vi "Create.vi"(8 "error in (no error)":errorcluster, 9 "# Chans":i32, 10 "Size":i32, 11 "MsgQ":refnum<class "MessageQ.lvclass">) -> (0 "error out":errorcluster, 3 "Data Buffer out":refnum<class "Data Buffer.lvclass">)   [LabVIEW 2020, in "VolatusData.lvlib" / "Data Buffer.lvclass"]
uses:
  Data Buffer.lvclass
  Data Buffer.lvclass/Data Buffer.ctl
  Volatus/MessageQ/MessageQ.lvclass
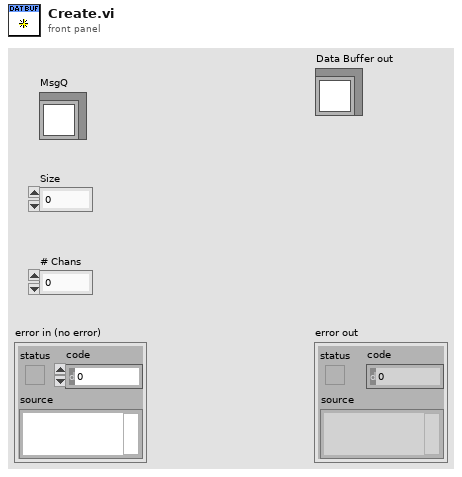
[diagram p1: front panel]
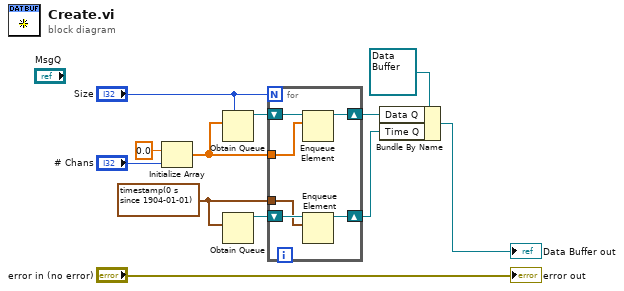
[diagram p0: block diagram]
diagram:
  w2 = timestamp(0 s since 1904-01-01)
  n1 = Initialize Array(0.0 ("element"), "# Chans") -> (w4:dbl[])
  n2 = Obtain Queue(max queue size (-1, unlimited)="Size", element data type=w4) -> (queue out=w9:refnum<queue>)  [unwired: 3 in, 2 out]
  n3 = Obtain Queue(element data type=w2) -> (queue out=w3:refnum<queue>)  [unwired: 4 in, 2 out]
  n4 = for {
    N: "Size" -> [_]
    shift-right: [w17] -> w6
    shift-left: w9 -> [w18]
    tunnel: w4 -> [w16]
    tunnel: w2 -> [w14]
    shift-right: [w13] -> w1
    shift-left: w3 -> [w15]
    n5 = Enqueue Element(queue=w18, element=w16) -> (queue out=w17:refnum<queue>)  [unwired: 2 in, 2 out]
    n6 = Enqueue Element(queue=w15, element=w14) -> (queue out=w13:refnum<queue>)  [unwired: 2 in, 2 out]
  }
  n7 = Bundle By Name(cluster=refnum<class "Data Buffer.lvclass"> refnum ("Data Buffer in"), "Data Q"=w6, "Time Q"=w1) -> (→"Data Buffer out":refnum<class "Data Buffer.lvclass">)
  "error out" <- "error in (no error)"
